vi "Run 4.vi"   [LabVIEW 2016]
types:
  T1 = typedef "LVHSConnector.ctl" = refnum<class "BrickReference.lvclass">
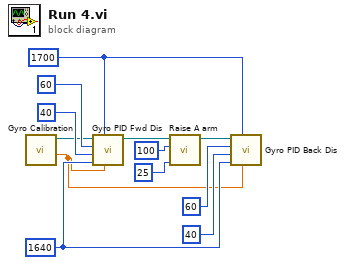
[diagram p0: block diagram]
diagram:
  w3 = 1640 ("Threshold to slow")
  w1 = 1700 ("Threshold to stop")
  n1 = call "Gyro Calibration.vi"() -> ("Degrees"=w2:sgl, "NXT/EV3"=w10:T1)  [unwired: 7 in, 1 out]
  n2 = call "Gyro PID Fwd Dis.vi"("Target angle"=w2, "Threshold to stop"=w1, "Threshold to slow"=w3, "Min. speed"=40, "Max. speed"=60, "EV3 in"=w10) -> ("EV3 out"=w9:T1)  [unwired: 5 in]
  n3 = call "Raise A arm.vi"("Power"=i8 25, "Rotation"=100, "EV3 in"=w9) -> ("EV3 out"=w6:T1)  [unwired: 8 in]
  n4 = call "Gyro PID Back Dis.vi"("Target angle"=w2, "Threshold to stop"=w1, "Threshold to slow"=w3, "Min. speed"=40, "Max. speed"=60, "EV3 in"=w6) -> ()  [unwired: 5 in, 1 out]
